vi "SingleButton BiStateVariableToggle.vi"(6 "AlreadySwitched?":bool, 9 "PreviousState":u16(ring) items=["State1", "State2"], 11 "Button":bool) -> (1 "NewState":u16(ring) items=["State1", "State2"], 4 "StillSwitched?":bool)   [LabVIEW 2017]
doc: "NOTE: USER OF THIS VI MUST ADD A FEEDBACK NODE CONNECTING THE \"StillSwitched?\" TERMINAL TO THE \"AlreadySwitched?\" TERMINAL.\nAllows switching the value of an enumerated GlobalVariable between two possible states. Each button press selects the alternate state."
panel:
  # "TODO: can put the feedback node internally\nbyRight click the VI Icon and go to VI Properties.\n Then select the category \"Execution\" and \nselect \"Preallocated clone reentrant execution\"."
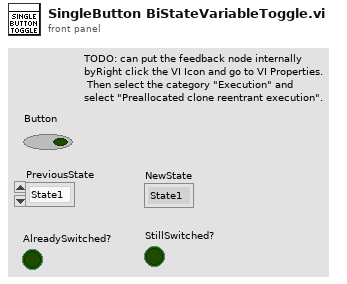
[diagram p1: front panel]
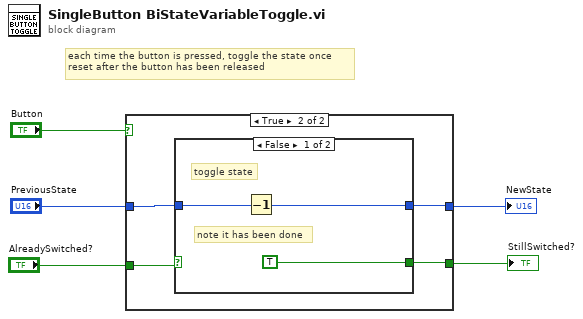
[diagram p0: block diagram]
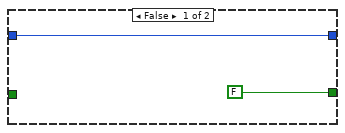
[diagram p2: hidden frame]
diagram:
  # "each time the button is pressed, toggle the state once \nreset after the button has been released"
  n1 = case shown="True" "Button" {
    tunnel: "PreviousState" -> [w7 w11]
    tunnel: [w7 w10] -> w3
    tunnel: "AlreadySwitched?" -> [_ w9]
    tunnel: [FALSE ("BiStateVariableToggle") w8] -> w1
    frame False {
    }
    frame True {
      n2 = case shown="False" w9 {
        selector: w9 -> [_ w15]
        tunnel: w11 -> [w14 w16]
        tunnel: [w13 w16] -> w10
        tunnel: [TRUE ("BiStateVariableSwitched") w15] -> w8
        frame False {
          # "note it has been done"
          # "toggle state"
          n3 = Decrement(x=w14) -> (x-1=w13:u16)
        }
        frame True {
          # "state has already been switched"
        }
      }
    }
  }
  "NewState" <- w3
  "StillSwitched?" <- w1
